vi "Config - SUM report - REPORT.vi"(4 "RVHR Cluster In":T1, 5 ".ini Controller":enum16{"Read", "Write"}(ring), 6 "End Time":timestamp, 7 ".ini filename":string="testconfiguration.ini", 8 "error in (no error)":errorcluster, 9 "Start Time":timestamp, 10 "Cluster in":T7 {"Settings Cluster"."Image Frequency" items=["2", "3", "5"]; "Settings Cluster"."Device Resolution" items=["0.1 µm", "1 µm", "10 µm"]; "Settings Cluster"."Distance Format" items=["kilometres", "miles & chains", "metres", "stations", "miles"]; "Settings Cluster"."Sampling Distance" items=["1mm", "2mm"]}, 11 "Directory Path":path) -> (0 "error out":errorcluster, 1 "Dates-Times":T6, 2 "Cluster out":T7 {"Settings Cluster"."Image Frequency" items=["2", "3", "5"]; "Settings Cluster"."Device Resolution" items=["0.1 µm", "1 µm", "10 µm"]; "Settings Cluster"."Distance Format" items=["kilometres", "miles & chains", "metres", "stations", "miles"]; "Settings Cluster"."Sampling Distance" items=["1mm", "2mm"]})   [LabVIEW 2023]
doc: "Obtains default hlc configuration information from an .ini file."
uses:
  <vilib>/Utility/config.llb/NI_LVConfig.lvlib
  Controls/SUM Cluster.ctl
  Controls/Test Cluster.ctl
  Controls/Distance Units.ctl
  Controls/Settings Cluster.ctl
  Controls/Sampling DIstance.ctl
  Controls/Device_Type.ctl
  Controls/Device_Resolution.ctl
  Controls/System information (YRCA - Truncate).ctl
  Controls/Run information (YRCA).ctl
  Controls/Run Description.ctl
  Controls/File Information CLuster.ctl
  Controls/Sum File Cluster (RCA).ctl
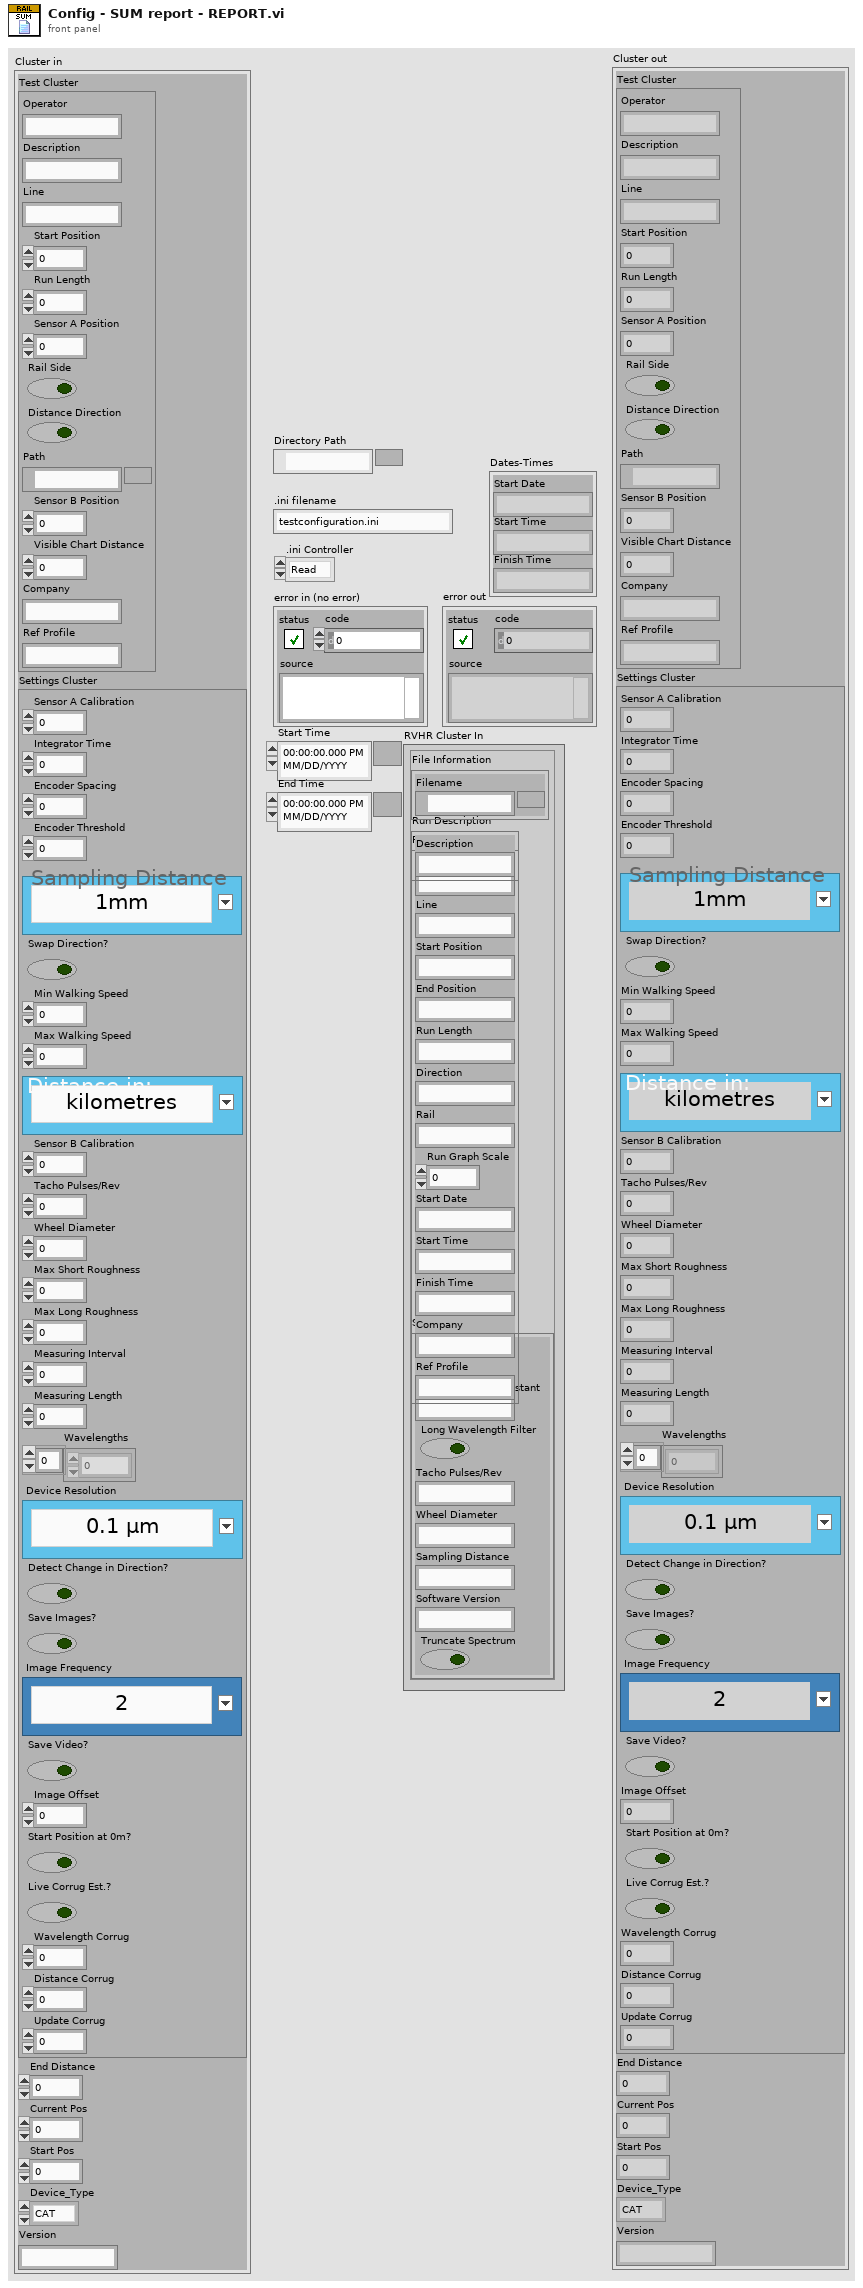
[diagram p1: front panel]
types:
  T1 = typedef "Sum File Cluster (RCA).ctl" = cluster{"File Information":T2, "Run Description":T3, "Run Information":T4, "System Information":T5}
  T2 = typedef "File Information CLuster.ctl" = cluster{"Filename":path}
  T3 = typedef "Run Description.ctl" = cluster{"Description":string}
  T4 = typedef "Run information (YRCA).ctl" = cluster{"Operator":string, "Line":string, "Start Position":string, "End Position":string, "Run Length":string, "Direction":string, "Rail":string, "Run Graph Scale":u16, "Start Date":string, "Start Time":string, "Finish Time":string, "Company":string, "Ref Profile":string}
  T5 = typedef "System information (YRCA - Truncate).ctl" = cluster{"Sensor Calibration":string, "Integrator Time Constant":string, "Long Wavelength Filter":bool, "Tacho Pulses/Rev":string, "Wheel Diameter":string, "Sampling Distance":string, "Software Version":string, "Truncate Spectrum":bool}
  T6 = cluster{"Start Date":string, "Start Time":string, "Finish Time":string}
  T7 = typedef "SUM Cluster.ctl" = cluster{"Test Cluster":T8, "Settings Cluster":T9, "End Distance":dbl, "Current Pos":dbl, "Start Pos":dbl, "Device_Type":T13, "Version":string}
  T8 = typedef "Test Cluster.ctl" = cluster{"Operator":string, "Description":string, "Line":string, "Start Position":dbl, "Run Length":dbl, "Sensor A Position":dbl, "Rail Side":bool, "Distance Direction":bool, "Path":path, "Sensor B Position":dbl, "Visible Chart Distance":dbl, "Company":string, "Ref Profile":string}
  T9 = typedef "Settings Cluster.ctl" = cluster{"Sensor A Calibration":dbl, "Integrator Time":dbl, "Encoder Spacing":dbl, "Encoder Threshold":dbl, "Sampling Distance":T10, "Swap Direction?":bool, "Min Walking Speed":dbl, "Max Walking Speed":dbl, "Distance Format":T11, "Sensor B Calibration":dbl, "Tacho Pulses/Rev":dbl, "Wheel Diameter":dbl, "Max Short Roughness":dbl, "Max Long Roughness":dbl, "Measuring Interval":dbl, "Measuring Length":dbl, "Wavelengths":dbl[], "Device Resolution":T12, "Detect Change in Direction?":bool, "Save Images?":bool, "Image Frequency":T10, "Save Video?":bool, "Image Offset":dbl, "Start Position at 0m?":bool, "Live Corrug Est.?":bool, "Wavelength Corrug":u8, "Distance Corrug":u8, "Update Corrug":u8}
  T10 = typedef "Sampling DIstance.ctl" = u16
  T11 = typedef "Distance Units.ctl" = u16
  T12 = typedef "Device_Resolution.ctl" = u16
  T13 = typedef "Device_Type.ctl" = enum16{"CAT", "Bi-CAT", "YRCA", "RCA", "RV-HR", "TV-HR"}
  T14 = typedef "NI_LVConfig.lvlib/Config Data RefNum.ctl" = refnum<k1>
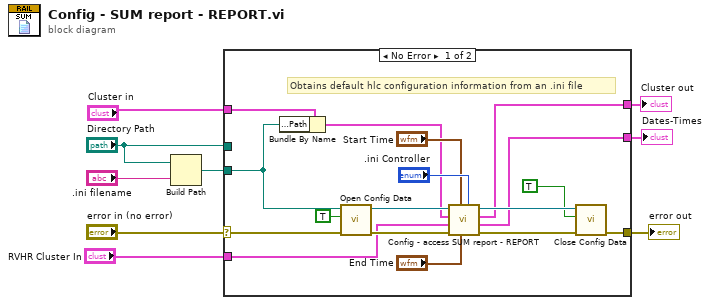
[diagram p0: block diagram]
diagram:
  n1 = Build Path(base path="Directory Path", name or relative path=".ini filename") -> (appended path=w7:path)
  n2 = case shown="No Error" "error in (no error)" {
    selector: "error in (no error)" -> [w16 w27]
    tunnel: [w20 _] -> w3
    tunnel: [w19 w27] -> w8
    tunnel: w7 -> [w12 _]
    tunnel: "Directory Path" -> [_ _]
    tunnel: "Cluster in" -> [w17 _]
    tunnel: [w11 _] -> w2
    tunnel: "RVHR Cluster In" -> [w10 _]
    frame No Error {
      # "Obtains default hlc configuration information from an .ini file"
      n3 = Bundle By Name(cluster=w17, "Test Cluster.Path"=w12) -> (w13:T7)
      n4 = call <vilib>:"Open Config Data.vi"("error in (no error)"=w16, "create file if necessary (T)"=TRUE, "configuration file path"=w12) -> ("error out"=w25:errorcluster, "refnum"=w23:T14)  [unwired: 6 in, 1 out]
      n5 = call "Config - access SUM report - REPORT.vi"(".ini Controller"=".ini Controller", "End Time"="End Time", "Start Time"="Start Time", "error in"=w25, "RVHR Cluster In"=w10, "Cluster in"=w13, "Config File Ref"=w23) -> ("error out"=w26:errorcluster, "Dates-Times"=w11:T6, "Cluster out"=w20:T7, "refnum out"=w24:T14)  [unwired: 1 in]
      n6 = call <vilib>:"Close Config Data.vi"("error in (no error)"=w26, "write file if changed (T)"=TRUE, "refnum"=w24) -> ("error out"=w19:errorcluster)  [unwired: 7 in, 1 out]
    }
    frame Error {
    }
  }
  "error out" <- w8
  "Cluster out" <- w3
  "Dates-Times" <- w2
